vi "2nd_ac_Vir_humid_air_2024.vi"(4 "CO2 content (ppm)":dbl=500.0, 5 "Type of air":i32(listbox)=4, 6 "xw molar fraction water vapor":dbl format="%.6g", 7 "Temperature (K)":dbl=300.0 format="%.4g") -> (0 "2nd ac pressure vir humid air b or \"F\"":dbl=6.3023779595165406e-09 format="%.2g", 1 "2nd ac vir humid air \"K\"":dbl=1.5720265750639378e-05 format="%.2e", 2 "2nd ac vir Water Kw":dbl=-0.0019546893543432725 format="%#_6e", 3 "2nd ac vir dry air Kd":dbl=1.5720265750639378e-05)   [LabVIEW 2016]
uses:
  SOS_Global_2022.vi
panel:
  out "2nd ac interaction vir air-water Kdw":dbl=-1.61224074030217e-05
  # "m^3 mol^-1"
  # "m^3 mol^-1"
  # "Pa^-1"
  # "m^3 mol^-1"
  # "m^3 mol^-1"
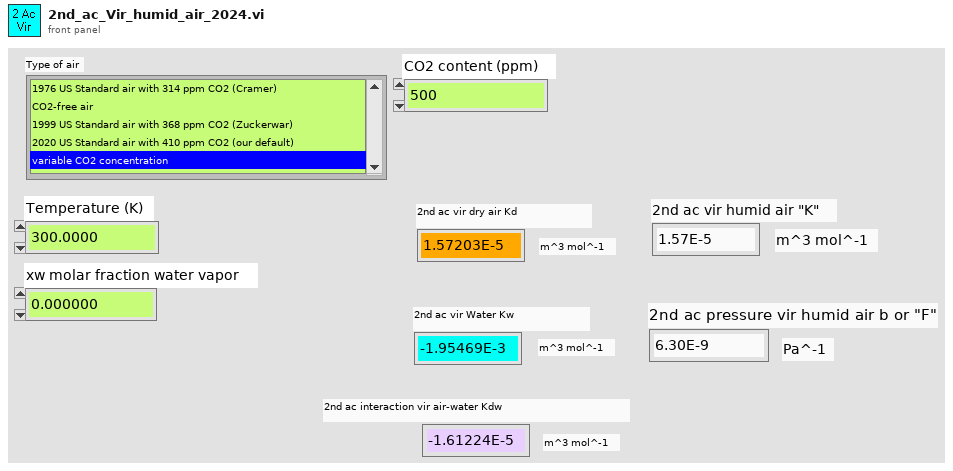
[diagram p1: front panel]
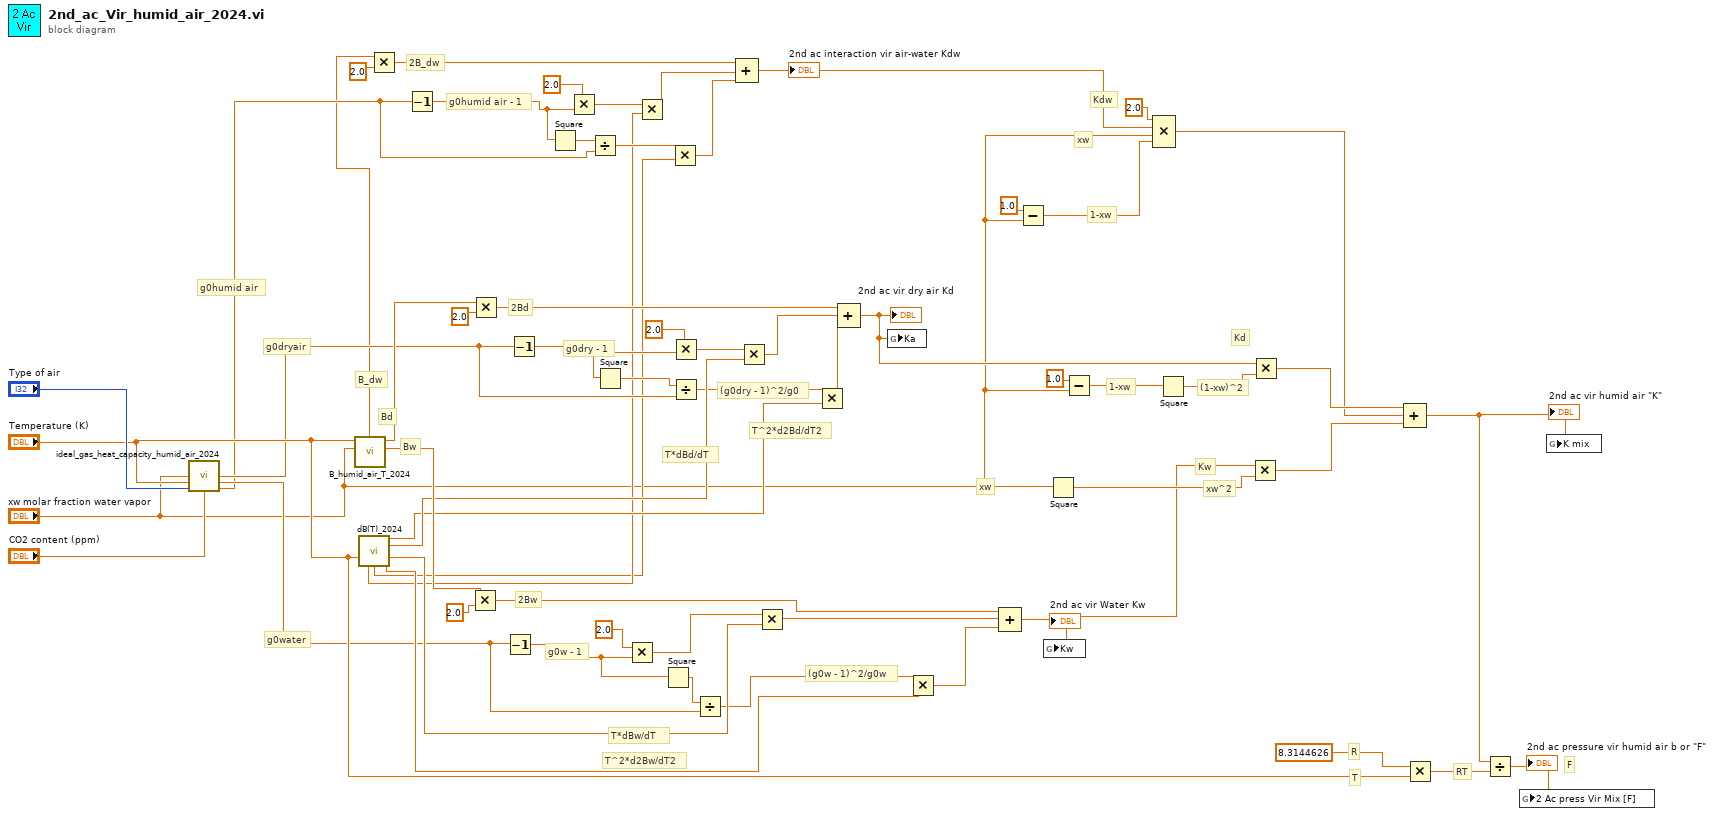
[diagram p0: block diagram]
diagram:
  # "g0humid air"
  # "(g0w - 1)^2/g0w"
  # "T^2*d2Bw/dT2"
  # "T*dBw/dT"
  # "T*dBd/dT"
  # "(g0dry - 1)^2/g0"
  # "T^2*d2Bd/dT2"
  # "RT"
  # "T"
  # "R"
  # "Kdw"
  # "xw^2"
  # "Kw"
  # "Kd"
  # "(1-xw)^2"
  # "1-xw"
  # "xw"
  # "1-xw"
  # "B_dw"
  # "g0humid air - 1"
  # "2B_dw"
  # "xw"
  # "g0w - 1"
  # "2Bw"
  # "Bw"
  # "g0dry - 1"
  # "Bd"
  # "2Bd"
  # "g0water"
  # "g0dryair"
  # "F"
  n1 = call "ideal_gas_heat_capacity_humid_air_2024.vi"("molar fraction of water vapor"="xw molar fraction water vapor", "Temperature [K]"="Temperature (K)", "Type of air"="Type of air", "CO2 content (ppm)"="CO2 content (ppm)") -> ("Gamma0 dry"=w23:dbl, "Gamma0 water"=w21:dbl, "Gamma0 humid air"=w9:dbl)  [unwired: 2 in, 7 out]
  n2 = call "B_humid_air_T_2024.vi"("xw molar fraction water vapor"="xw molar fraction water vapor", "Temperature (K)"="Temperature (K)") -> ("Bdw(T) [m^3/mol]"=w8:dbl, "Bw(T) [m^3/mol]"=w42:dbl, "Bd(T) [m^3/mol]"=w43:dbl)  [unwired: 5 in, 2 out]
  n3 = call "dB(T)_2024.vi"("Temperature (K)"="Temperature (K)") -> ("T^2*d^2Bair/dT^2"=w35:dbl, "T*dBair/dT"=w38:dbl, "T*dBwater/dT"=w31:dbl, "T^2*d^2Bwater/dT^2"=w28:dbl, "T^2*d^2Bair-water/dT^2"=w5:dbl, "T*dBair-water/dT"=w6:dbl)  [unwired: 3 in, 6 out]
  n4 = Multiply(x=w8, y=2.0) -> (x*y=w17:dbl)
  n5 = Decrement(x=w9) -> (x-1=w10:dbl)
  n6 = Multiply(x=w42, y=2.0) -> (x*y=w54:dbl)
  n7 = Multiply(x=w43, y=2.0) -> (x*y=w55:dbl)
  n8 = Decrement(x=w21) -> (x-1=w20:dbl)
  n9 = Decrement(x=w23) -> (x-1=w22:dbl)
  n10 = Square(x=w10) -> (x^2=w13:dbl)
  n11 = Multiply(x=2.0, y=w10) -> (x*y=w15:dbl)
  n12 = Divide(x=w13, y=w9) -> (x/y=w12:dbl)
  n13 = Square(x=w22) -> (x^2=w36:dbl)
  n14 = Multiply(x=2.0, y=w20) -> (x*y=w32:dbl)
  n15 = Multiply(x=w15, y=w6) -> (x*y=w14:dbl)
  n16 = Square(x=w20) -> (x^2=w56:dbl)
  n17 = Multiply(x=w12, y=w5) -> (x*y=w11:dbl)
  n18 = Multiply(x=2.0, y=w22) -> (x*y=w39:dbl)
  n19 = Divide(x=w36, y=w23) -> (x/y=w34:dbl)
  n20 = Divide(x=w56, y=w21) -> (x/y=w29:dbl)
  n21 = Compound Arithmetic op=ADD(w17, w14, w11) -> (w4:dbl)
  "2nd ac interaction vir air-water Kdw" <- w4
  n22 = Multiply(x=w39, y=w38) -> (x*y=w37:dbl)
  n23 = Multiply(x=w32, y=w31) -> (x*y=w30:dbl)
  n24 = Multiply(x=w34, y=w35) -> (x*y=w33:dbl)
  n25 = Compound Arithmetic op=ADD(w55, w37, w33) -> (w26:dbl)
  "2nd ac vir dry air Kd" <- w26
  n26 = global write "SOS_Global_2022.vi" "Ka"(w26) -> ()
  n27 = Multiply(x=w29, y=w28) -> (x*y=w27:dbl)
  n28 = Compound Arithmetic op=ADD(w54, w30, w27) -> (w25:dbl)
  "2nd ac vir Water Kw" <- w25
  n29 = Subtract(x=1.0, y="xw molar fraction water vapor") -> (x-y=w1:dbl)
  n30 = global write "SOS_Global_2022.vi" "Kw"(w25) -> ()
  n31 = Square(x="xw molar fraction water vapor") -> (x^2=w50:dbl)
  n32 = Subtract(x=1.0, y="xw molar fraction water vapor") -> (x-y=w52:dbl)
  n33 = Compound Arithmetic op=MULTIPLY(2.0 ("value"), w4, "xw molar fraction water vapor", w1) -> (w7:dbl)
  n34 = Square(x=w52) -> (x^2=w51:dbl)
  n35 = Multiply(x=w25, y=w50) -> (x*y=w48:dbl)
  n36 = Multiply(x=w26, y=w51) -> (x*y=w49:dbl)
  n37 = Compound Arithmetic op=ADD(w49, w7, w48) -> (w45:dbl)
  "2nd ac vir humid air \"K\"" <- w45
  n38 = Multiply(x=8.3144626, y="Temperature (K)") -> (x*y=w47:dbl)
  n39 = Divide(x=w45, y=w47) -> (x/y=w44:dbl)
  "2nd ac pressure vir humid air b or \"F\"" <- w44
  n40 = global write "SOS_Global_2022.vi" "2 Ac press Vir Mix [F]"(w44) -> ()
  n41 = global write "SOS_Global_2022.vi" "K mix"(w45) -> ()
